vi "Is Error.vi"(8 "error in (no error)":errorcluster, 11 "error":T1=enum."Out of Bounds") -> (0 "error out":errorcluster, 3 "is error?":bool)   [LabVIEW 2020, in "Memory Manager.lvlib" / "Pointer.lvclass"]
uses:
  Pointer.lvclass
  Errors.ctl
  Pointer.lvclass/Pointer.ctl
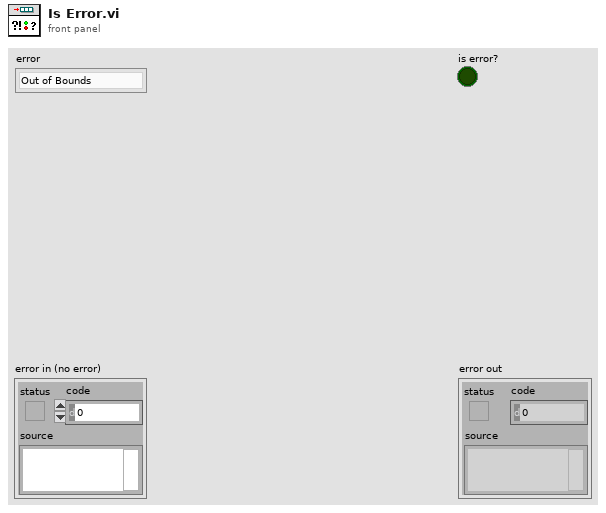
[diagram p1: front panel]
types:
  T1 = typedef "Memory Manager.lvlib/Pointer.lvclass/Errors.ctl" = enum16{"No Error", "Null Pointer", "Out of Bounds", "Buffer Underflow", "Size Mismatch", "Zone"}
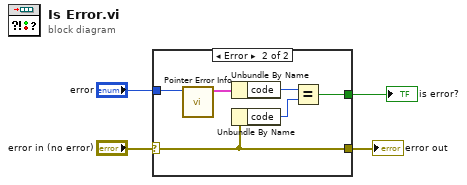
[diagram p0: block diagram]
diagram:
  n1 = case shown="Error" "error in (no error)" {
    selector: "error in (no error)" -> [w5 w11]
    tunnel: [w5 w11] -> w3
    tunnel: "error" -> [_ w10]
    tunnel: [_ w6] -> w1
    frame No Error {
    }
    frame Error {
      n2 = call "Pointer Error Info.vi"("error"=w10) -> ("error info"=w9:cluster{"code":i32, "description":string})  [unwired: 10 in]
      n3 = Unbundle By Name(w9) -> ("code"=w8:i32)
      n4 = Unbundle By Name(w11) -> ("code"=w7:i32)
      n5 = Equal?(x=w8, y=w7) -> (x = y?=w6:bool)
    }
  }
  "error out" <- w3
  "is error?" <- w1
